vi "NT Read and Format as String.vi"(11 "Name":string="Boolean") -> (3 "Formatted String":string)   [LabVIEW 2020]
doc: "Read the named network table entry and return the data formatted as a string."
panel:
  in  "error in":errorcluster
  out "error out":errorcluster
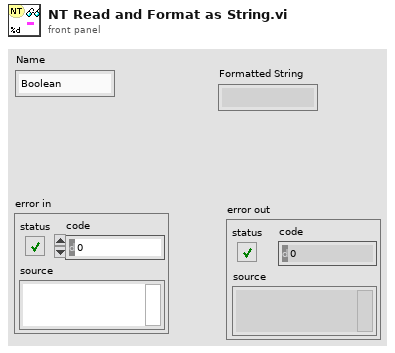
[diagram p1: front panel]
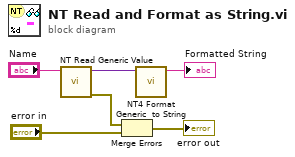
[diagram p0: block diagram]
diagram:
  n1 = call "NT Read Generic Value.vi"("name"="Name") -> ("error out"=w4:errorcluster, "variant value"=w2:variant)  [unwired: 9 in]
  n2 = Merge Errors(w4, "error in") -> (→"error out":errorcluster)
  n3 = call "NT4 Format Generic  to String.vi"("Variant"=w2) -> ("String"=→"Formatted String":string)  [unwired: 9 in, 1 out]
